vi "Enum to Gain.vi"(1 "Gain":T1) -> (0 "Gain (x)":dbl)   [LabVIEW 2019, in "KH7008.lvlib"]
uses:
  KH7008.lvlib
  Inst.Krohn-Hite-7008/Typedefs/Gain-Enum.ctl
  <userlib>/LevyLab/Instrument Framework/SMOs/Instrument/Instrument.lvclass
  Inst.Krohn-Hite-7008/Inst.Krohn-Hite-7008.lvclass
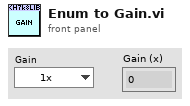
[diagram p1: front panel]
types:
  T1 = typedef "Inst.Krohn-Hite-7008.lvclass/Gain-Enum.ctl" = enum16{"1x", "10x", "100x", "1000x"}
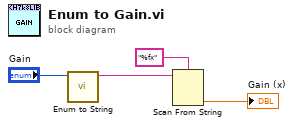
[diagram p0: block diagram]
diagram:
  n1 = call <userlib>:"Enum to String.vi"("Command"="Gain") -> ("Command"=w3:string)  [unwired: 9 in, 1 out]
  n2 = Scan From String(format string="%fx", input string=w3) -> (output 1=→"Gain (x)":dbl)  [unwired: 3 in, 3 out]
